vi "Close references.vi"(0 "LV DEV in":refnum<class "LV DEV.lvclass">, 11 "error in (no error)":errorcluster) -> (4 "LV DEV out":refnum<class "LV DEV.lvclass">, 15 "error out":errorcluster)   [LabVIEW 2016, in "LV DEV.lvclass"]
uses:
  LV DEV.lvclass
  D:/MDI Project/source code/Document/LV Doc/LV Doc.lvclass
  LV DEV.lvclass/LV DEV.ctl
  LV Doc.lvclass/LV Doc.ctl
  property/Read application reference.vi
  property/Read VI Reference.vi
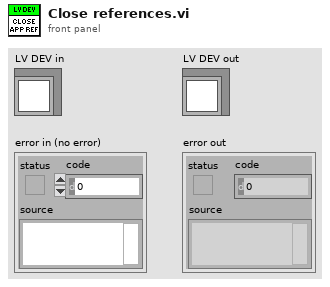
[diagram p1: front panel]
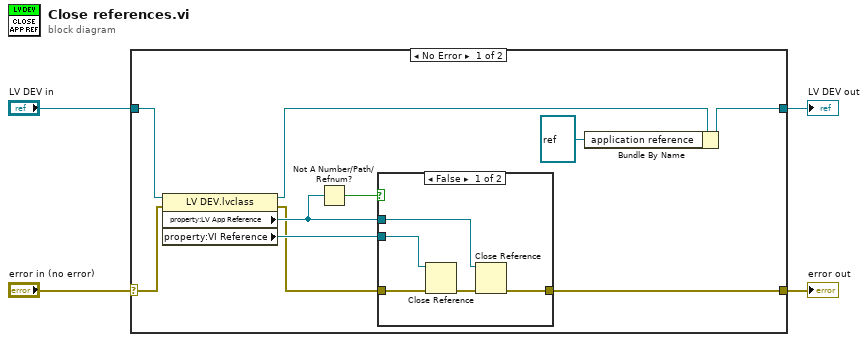
[diagram p0: block diagram]
diagram:
  n1 = case shown="No Error" "error in (no error)" {
    selector: "error in (no error)" -> [w8 w22]
    tunnel: [w14 w22] -> w3
    tunnel: [w13 w21] -> w1
    tunnel: "LV DEV in" -> [w6 w21]
    frame No Error {
      n2 = property class="LV DEV.lvclass"(reference=w6, error in=w8) -> (reference out=w5:refnum<class "LV DEV.lvclass">, error out=w7:errorcluster, "property:LV App Reference"=w10:refnum<vi>, "property:VI Reference"=w9:refnum<vi>)
      n3 = Not A Number/Path/Refnum?(number/path/refnum=w10) -> (NaN/Path/Refnum?=w11:bool)
      n4 = case shown="False" w11 {
        tunnel: w7 -> [w16 w20]
        tunnel: [w19 w20] -> w14
        tunnel: w10 -> [w18 _]
        tunnel: w9 -> [w17 _]
        frame False {
          n5 = Close Reference(reference=w17, error in (no error)=w16) -> (error out=w15:errorcluster)
          n6 = Close Reference(reference=w18, error in (no error)=w15) -> (error out=w19:errorcluster)
        }
        frame True {
        }
      }
      n7 = Bundle By Name(cluster=w5, "application reference"=refnum<vi> refnum) -> (w13:refnum<class "LV DEV.lvclass">)
    }
    frame Error {
    }
  }
  "error out" <- w3
  "LV DEV out" <- w1
